vi "Read Log.vi"(8 "error in (no error)":errorcluster, 10 "Log Path":path, 11 "DBLayout in":refnum<class "DBLayout.lvclass">) -> (0 "error out":errorcluster, 2 "Log":string, 3 "DBLayout out":refnum<class "DBLayout.lvclass">)   [LabVIEW 2019, in "TSC Event Logger (SQL).lvlib" / "DBLayout.lvclass"]
uses:
  DBLayout.lvclass
  <vilib>/drjdpowell/SQLite Library/SQL Connection/Open (path).vi
  <vilib>/drjdpowell/SQLite Library/SQL Connection/Open (string).vi
  <vilib>/AdvancedString/Path To Command Line String.vi
  <vilib>/drjdpowell/SQLite Library/SQL Connection/Execute SQL.vi
  <vilib>/drjdpowell/SQLite Library/SQL Connection/Connection.lvclass
  <vilib>/drjdpowell/SQLite Library/SQLite.lvlib
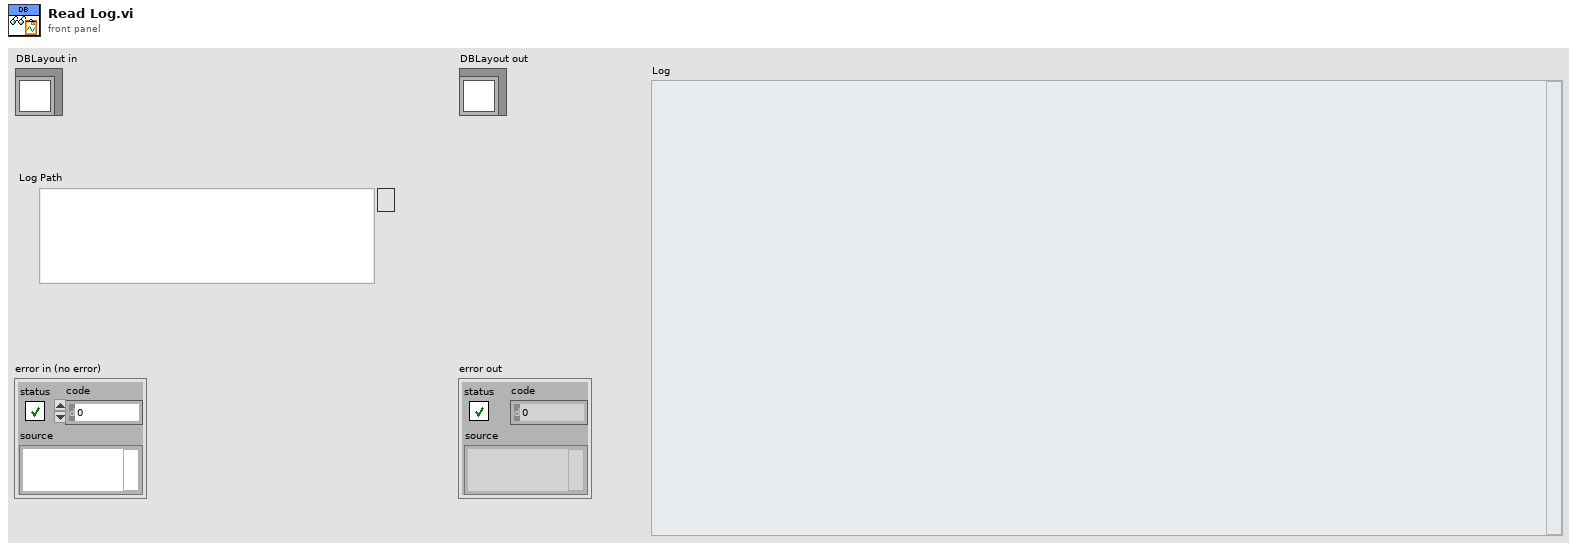
[diagram p1: front panel]
types:
  T1 = enum16{"New or existing", "Existing", "Read only"}
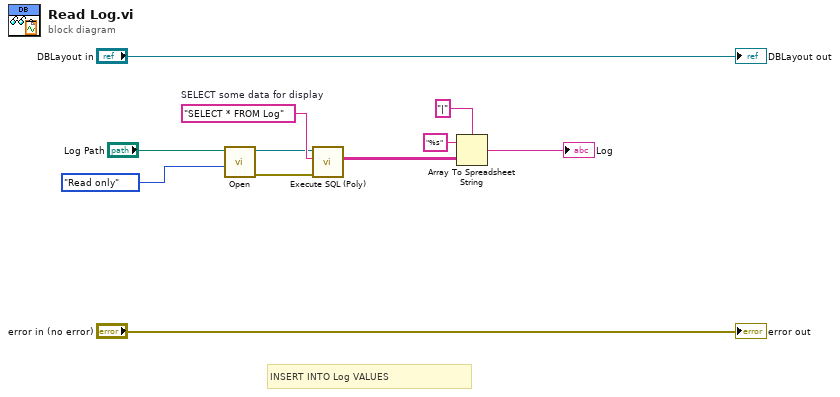
[diagram p0: block diagram]
diagram:
  w7 = "SELECT * FROM Log"  # SELECT some data for display
  # "INSERT INTO Log VALUES"
  n1 = call-poly <vilib>:"Open.vi"("File Option"=T1."Read only", "db file"="Log Path") -> ("error out"=w5:errorcluster, "SQLite Connection"=w6:refnum<class "Connection.lvclass">)  [unwired: 8 in]
  n2 = call-poly <vilib>:"Execute SQL (Poly).vi"("error in (no error)"=w5, "SQL"=w7, "SQLite Connection in"=w6) -> ("Result Set"=w4:string[][])  [unwired: 5 in, 3 out]
  n3 = Array To Spreadsheet String(delimiter (Tab)="|", array=w4, 3:"%s" ("format string")) -> (spreadsheet string=→"Log":string)
  "error out" <- "error in (no error)"
  "DBLayout out" <- "DBLayout in"
